vi "Apply Language.vi"(8 "error in (no error)":errorcluster, 11 "Controller in":refnum<class "Controller.lvclass">) -> (0 "error out":errorcluster, 3 "Controller out":refnum<class "Controller.lvclass">)   [LabVIEW 2013, in "SET Project Editor.lvlib" / "Controller.lvclass"]
uses:
  Controller.lvclass
  Wizards/Apply Language Wizard/Apply Language Wizard.lvclass
  Controller.lvclass/Controller.ctl
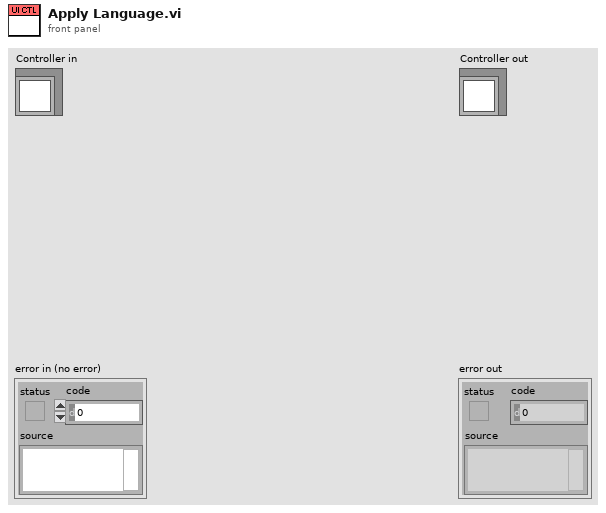
[diagram p1: front panel]
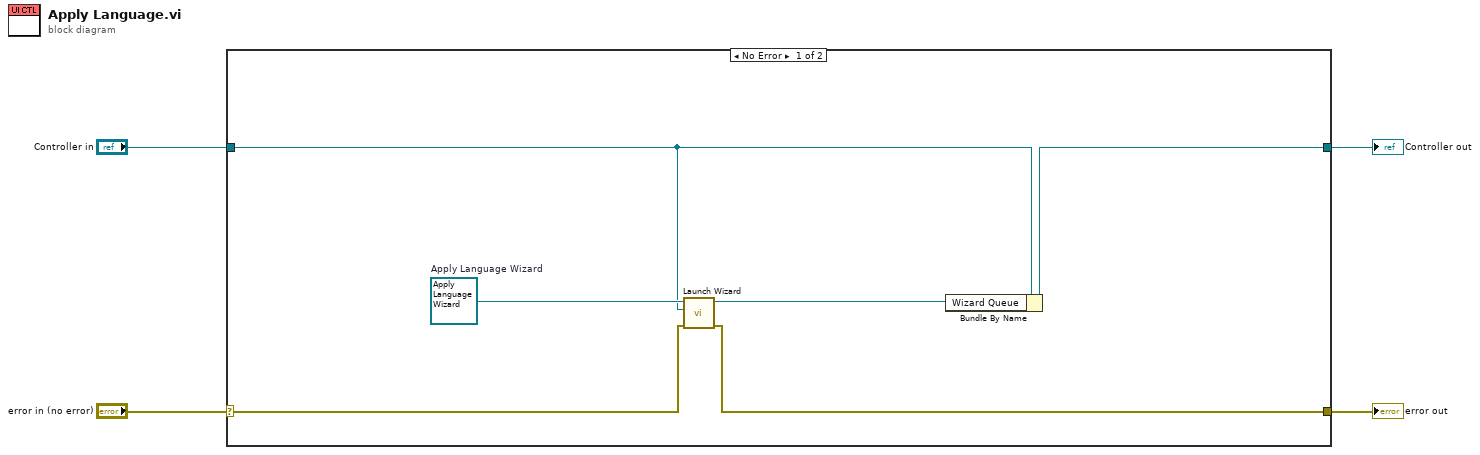
[diagram p0: block diagram]
diagram:
  n1 = case shown="No Error" "error in (no error)" {
    selector: "error in (no error)" -> [w8 w12]
    tunnel: [w10 w12] -> w3
    tunnel: [w9 w11] -> w1
    tunnel: "Controller in" -> [w5 w11]
    frame No Error {
      w6 = refnum<class "Apply Language Wizard.lvclass"> refnum  # Apply Language Wizard
      n2 = call-dynamic "Launch Wizard.vi"("error in (no error)"=w8, "Controller in"=w5, "UI Wizard in"=w6) -> ("error out"=w10:errorcluster, "Caller-To-Actor Enqueuer"=w7:refnum<class "Message Enqueuer.lvclass">)  [unwired: 7 in]
      n3 = Bundle By Name(cluster=w5, "Wizard Queue"=w7) -> (w9:refnum<class "Controller.lvclass">)
    }
    frame Error {
    }
  }
  "error out" <- w3
  "Controller out" <- w1
